vi "Config Scan Sample.vi"(0 "VISA resource name":refnum<visa-resource-name>, 1 "Coupling (0)":i32 min=0 max=3, 2 "Floor (1)":i32=1 min=1 max=8, 3 "Ceiling (8)":i32=8 min=1 max=8, 4 "Method (discrete)":enum16{"discrete"}(ring), 5 "Method Value (1)":i32(ring)=1 items=["-1"=-1, "1"=1], 7 "error in":errorcluster) -> (20 "VISA resource name out":refnum<visa-resource-name>, 27 "error out":errorcluster)   [LabVIEW 2019, in "Andeen-Hagerling 2700(400 firmware).lvlib"]
doc: "Establishes the position of sample switch scanning within the multidimensional parameter scanning system. Also sets the highest and lowest sample switch numbers to be used during scanning. and the direction in which the sample number is changed each time a scan measurement is to be taken."
uses:
  Andeen-Hagerling 2700(400 firmware).lvlib
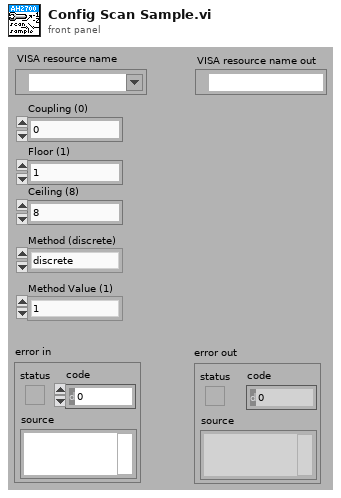
[diagram p1: front panel]
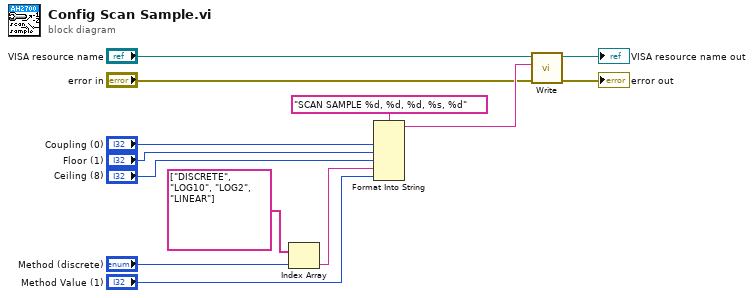
[diagram p0: block diagram]
diagram:
  n1 = Index Array(array=string[] ["DISCRETE", "LOG10", "LOG2", "LINEAR"], index="Method (discrete)") -> (element=w1:string)
  n2 = Format Into String(format string="SCAN SAMPLE %d, %d, %d, %s, %d", "Coupling (0)", "Floor (1)", "Ceiling (8)", w1, "Method Value (1)") -> (resulting string=w11:string)  [unwired: 2 in, 1 out]
  n3 = call "Write.vi"("error in"="error in", "command"=w11, "VISA resource name"="VISA resource name") -> ("error out"=→"error out":errorcluster, "VISA resource name out"=→"VISA resource name out":refnum<visa-resource-name>)  [unwired: 7 in]
